vi "Get LogicIO Labels.vi"(8 "error in (no error)":errorcluster, 11 "VacuumLine in":refnum<class "VacuumLine.lvclass">) -> (0 "error out":errorcluster, 2 "LogicIO Labels":string[](array[string]), 3 "VacuumLine out":refnum<class "VacuumLine.lvclass">)   [LabVIEW 2016, in "Hardware.lvlib" / "VacuumLine.lvlib" / "VacuumLine.lvclass"]
uses:
  <userlib>/Common Components/Hardware/Abstract System/VacuumLine/VacuumLine/VacuumLine.lvclass
  <userlib>/Common Components/Hardware/Abstract System/VacuumLine/VacuumLine/VacuumLine.lvclass/VacuumLine.ctl
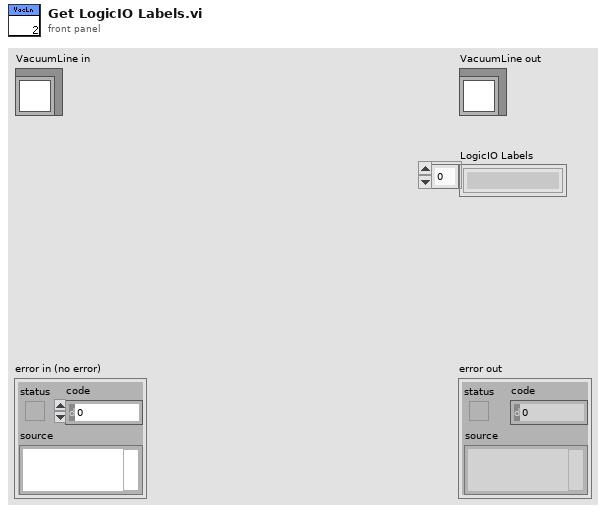
[diagram p1: front panel]
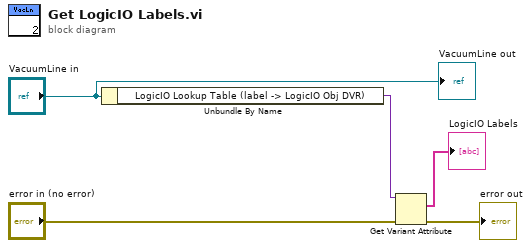
[diagram p0: block diagram]
diagram:
  n1 = Unbundle By Name("VacuumLine in") -> ("LogicIO Lookup Table (label -> LogicIO Obj DVR)"=w4:variant)
  n2 = Get Variant Attribute(Variant=w4, error in="error in (no error)") -> (names=→"LogicIO Labels":string[], error out=→"error out":errorcluster)  [unwired: 2 in, 2 out]
  "VacuumLine out" <- "VacuumLine in"
